vi "Initialization(SubVI for PI).vi"() -> (0 "error out":errorcluster, 3 "Position":dbl[](array[numeric])=[5.001098633, 3.755004883, 6.394439697])   [LabVIEW 2020]
uses:
  Global Parameters.vi
panel:
  in  "USB settings":cluster{"S/N":string, "USB Search?":bool}={"S/N"="0120020544", "USB Search?"=FALSE}
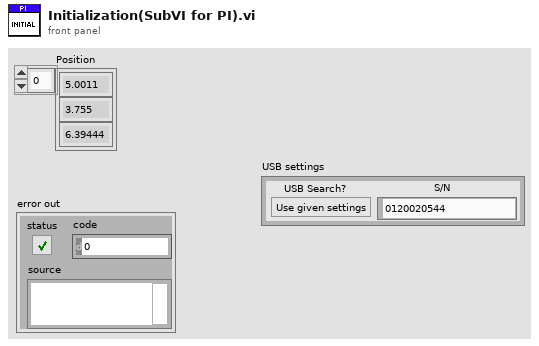
[diagram p1: front panel]
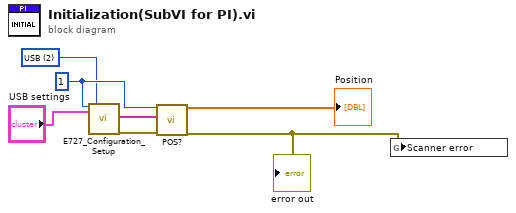
[diagram p0: block diagram]
diagram:
  w3 = u16 2 items=["RS232", "TCP/IP", "USB"] ("Interface")
  w4 = 1 ("System no.")
  n1 = call "E727_Configuration_Setup.vi"("System no."=w4, "USB settings"="USB settings", "Interface"=w3) -> ("All conn. axes"=w5:string[], "error out"=w7:errorcluster)  [unwired: 11 in, 4 out]
  n2 = call "POS?.vi"("System no."=w4, "Axes to query"=w5, "error in"=w7) -> ("Position"=→"Position":dbl[], "error out"=w2:errorcluster)  [unwired: 2 in, 13 out]
  "error out" <- w2
  n3 = global write "Global Parameters.vi" "Scanner error"(w2) -> ()
